vi "Handle Tree Shortcut Selection Event.vi"(6 "coords":T1, 8 "error in":errorcluster, 9 "tree refnum":refnum<vi>, 10 "ItemTag":string, 11 "state in":T2) -> (0 "error out":errorcluster, 2 "update tree?":bool, 3 "state out":T2)   [LabVIEW 2010, in "NI_SE_Config Front Panel Layout.lvlib"]
uses:
  NI_SE_Config Front Panel Layout.lvlib
  State.ctl
  VI Info.ctl
  VI Panel Layout/VI Panel Layout.lvclass
  <vilib>/Utility/miscctls.llb/LVPoint32TypeDef.ctl
  Get VI Info Index by Name.vi
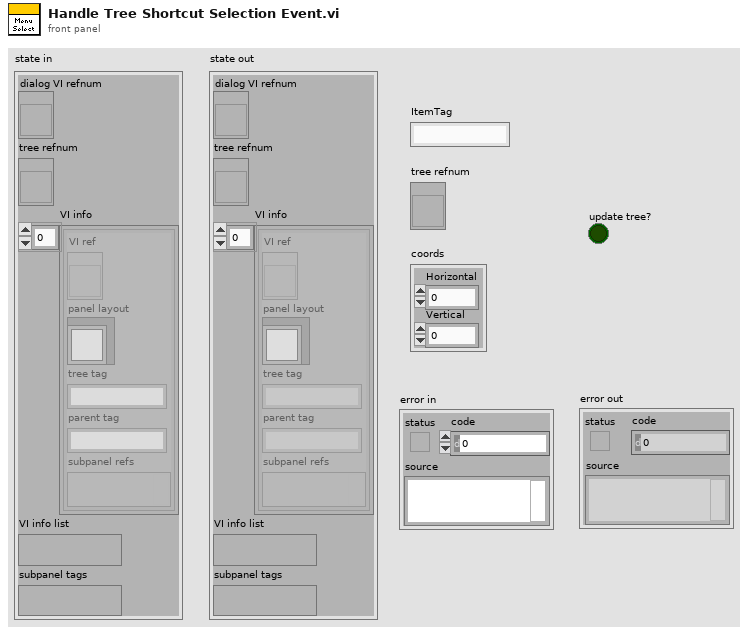
[diagram p1: front panel]
types:
  T1 = typedef "LVPoint32TypeDef.ctl" = cluster{"Horizontal":i32, "Vertical":i32}
  T2 = typedef "NI_SE_Config Front Panel Layout.lvlib/State.ctl" = cluster{"dialog VI refnum":refnum<vi>, "tree refnum":refnum<vi>, "VI info":T3[], "VI info list":variant, "subpanel tags":variant}
  T3 = typedef "NI_SE_Config Front Panel Layout.lvlib/VI Info.ctl" = cluster{"VI ref":refnum<vi>, "panel layout":refnum<class "VI Panel Layout.lvclass">, "tree tag":string, "parent tag":string, "subpanel refs":variant}
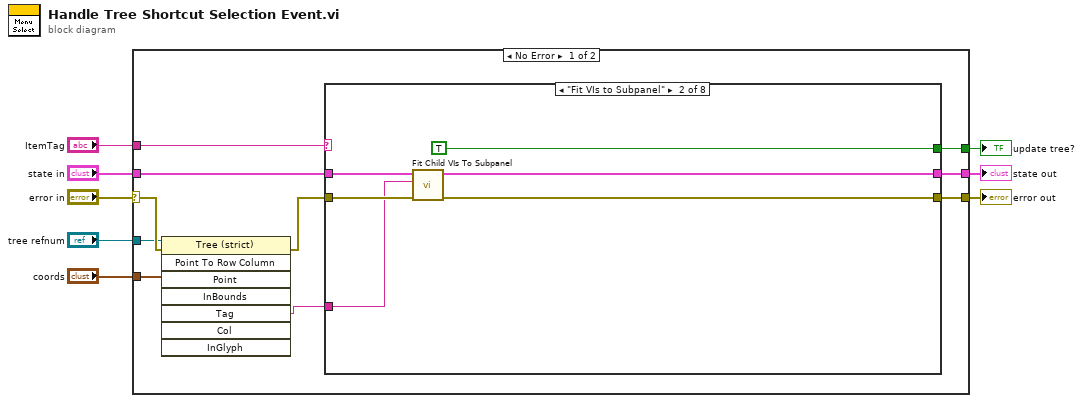
[diagram p0: block diagram]
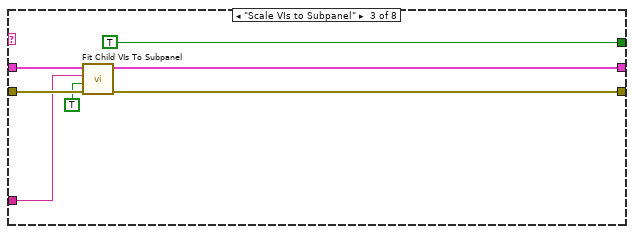
[diagram p3: hidden frame]
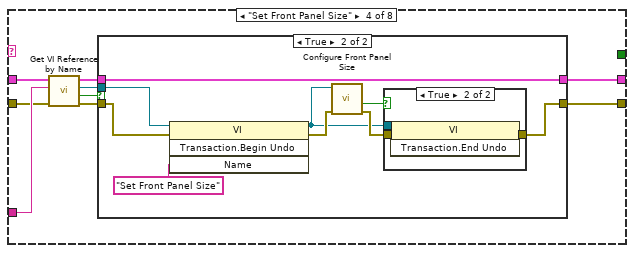
[diagram p4: hidden frame]
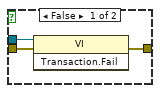
[diagram p6: hidden frame]
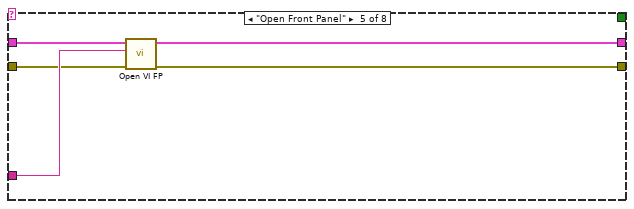
[diagram p7: hidden frame]
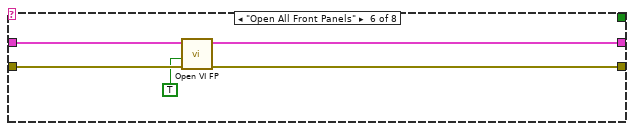
[diagram p8: hidden frame]
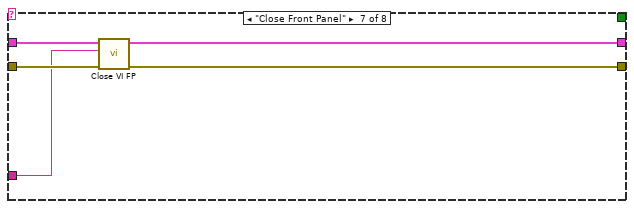
[diagram p9: hidden frame]
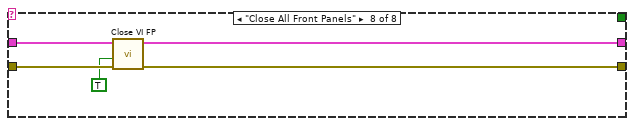
[diagram p10: hidden frame]
diagram:
  n1 = case shown="No Error" "error in" {
    selector: "error in" -> [w15 w80]
    tunnel: "state in" -> [w16 w81]
    tunnel: [w10 w81] -> w6
    tunnel: [w11 w80] -> w5
    tunnel: "tree refnum" -> [w14 _]
    tunnel: "coords" -> [w13 _]
    tunnel: "ItemTag" -> [w12 _]
    tunnel: [w9 _] -> w1
    frame No Error {
      n2 = invoke class="Tree (strict)" method="Point To Row Column"(reference=w14, error in=w15, "Point"=w13) -> (error out=w18:errorcluster, "Tag"=w17:string)  [unwired: 5 in, 6 out]
      n3 = case shown="\"Fit VIs to Subpanel\"" w12 {
        tunnel: w16 -> [w20 w26 w33 w42 w64 w69 w74 w79]
        tunnel: [w20 w24 w31 w35 w63 w67 w73 w78] -> w10
        tunnel: w18 -> [w19 w25 w32 w40 w60 w68 w72 w77]
        tunnel: [w19 w23 w30 w36 w62 w66 w71 w76] -> w11
        tunnel: w17 -> [_ w22 w29 w41 w61 _ w70 _]
        tunnel: [_ TRUE TRUE _ _ _ _ _] -> w9
        frame Default {
        }
        frame "Fit VIs to Subpanel" {
          n4 = call "Fit Child VIs To Subpanel.vi"("error in"=w25, "subpanel tag"=w22, "state in"=w26) -> ("error out"=w23:errorcluster, "state out"=w24:T2)  [unwired: 7 in]
        }
        frame "Scale VIs to Subpanel" {
          n5 = call "Fit Child VIs To Subpanel.vi"("error in"=w32, "scale VI layouts? (F)"=TRUE, "subpanel tag"=w29, "state in"=w33) -> ("error out"=w30:errorcluster, "state out"=w31:T2)  [unwired: 6 in]
        }
        frame "Set Front Panel Size" {
          n6 = call "Get VI Reference by Name.vi"("error in"=w40, "VI name"=w41, "state in"=w42) -> ("error out"=w38:errorcluster, "found?"=w39:bool, "VI ref"=w34:refnum<vi>, "state out"=w37:T2)  [unwired: 5 in]
          n7 = case shown="True" w39 {
            tunnel: w38 -> [w44 w52]
            tunnel: w37 -> [w43 w53]
            tunnel: [w44 w48] -> w36
            tunnel: [w43 w53] -> w35
            tunnel: w34 -> [_ w46]
            frame False {
            }
            frame True {
              n8 = invoke class="VI" method="Transaction.Begin Undo"(reference=w46, error in=w52, "Name"="Set Front Panel Size") -> (reference out=w45:refnum<vi>, error out=w51:errorcluster)  [unwired: 1 in, 2 out]
              n9 = call "Configure Front Panel Size.vi"("error in"=w51, "VI ref"=w45) -> ("error out"=w49:errorcluster, "applied"=w47:bool)  [unwired: 8 in]
              n10 = case shown="True" w47 {
                tunnel: w45 -> [w56 w59]
                tunnel: w49 -> [w55 w58]
                tunnel: [w54 w57] -> w48
                frame False {
                  n11 = invoke class="VI" method="Transaction.Fail"(reference=w56, error in=w55) -> (error out=w54:errorcluster)  [unwired: 1 in, 2 out]
                }
                frame True {
                  n12 = invoke class="VI" method="Transaction.End Undo"(reference=w59, error in=w58) -> (error out=w57:errorcluster)  [unwired: 1 in, 2 out]
                }
              }
            }
          }
        }
        frame "Open Front Panel" {
          n13 = call "Open VI FP.vi"("error in"=w60, "VI name"=w61, "state in"=w64) -> ("error out"=w62:errorcluster, "state out"=w63:T2)  [unwired: 7 in]
        }
        frame "Open All Front Panels" {
          n14 = call "Open VI FP.vi"("error in"=w68, "open all VI panels? (F)"=TRUE, "state in"=w69) -> ("error out"=w66:errorcluster, "state out"=w67:T2)  [unwired: 7 in]
        }
        frame "Close Front Panel" {
          n15 = call "Close VI FP.vi"("error in"=w72, "VI name (\"\")"=w70, "state in"=w74) -> ("error out"=w71:errorcluster, "state out"=w73:T2)  [unwired: 7 in]
        }
        frame "Close All Front Panels" {
          n16 = call "Close VI FP.vi"("error in"=w77, "close all VI panels? (F)"=TRUE, "state in"=w79) -> ("error out"=w76:errorcluster, "state out"=w78:T2)  [unwired: 7 in]
        }
      }
    }
    frame Error {
    }
  }
  "state out" <- w6
  "error out" <- w5
  "update tree?" <- w1
